vi "swingup_pendulum_energy.vi"(0 "alpha_full (rad)":dbl, 1 "alpha_dot (rad/s)":dbl, 2 "mp (kg)":dbl=0.027000000700354576 caption="Mp" min=0.0 step=0.0010000000474974513 format="%_3f", 3 "lp (m)":dbl=0.15299999713897705 caption="lp" min=0.0 max=1.0 step=0.0010000000474974513 format="%#_3f", 4 "Jp (kg.m^2)":dbl=0.00011999999696854502 caption="Jp" min=0.0 max=0.0010000000474974513 step=9.999999747378752e-06 format="%_3g") -> (5 "E (mJ)":dbl)   [LabVIEW 2021]
doc: "Calculates the total energy of a pendulum."
panel:
  # "Distance from pivot to CM"
  # "Moment of inertia about CM."
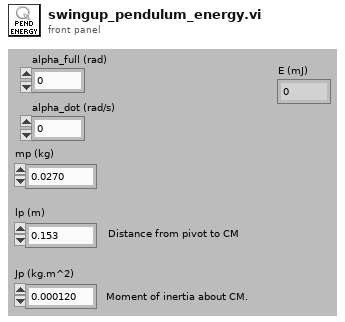
[diagram p1: front panel]
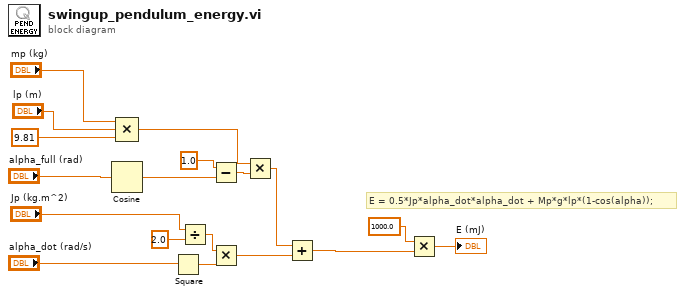
[diagram p0: block diagram]
diagram:
  # "E = 0.5*Jp*alpha_dot*alpha_dot + Mp*g*lp*(1-cos(alpha));"
  n1 = Cosine(x="alpha_full (rad)") -> (cos(x)=w11:dbl)
  n2 = Compound Arithmetic op=MULTIPLY("mp (kg)", "lp (m)", 9.81 ("value")) -> (w12:dbl)
  n3 = Square(x="alpha_dot (rad/s)") -> (x^2=w18:dbl)
  n4 = Divide(x="Jp (kg.m^2)", y=2.0) -> (x/y=w17:dbl)
  n5 = Subtract(x=1.0, y=w11) -> (x-y=w14:dbl)
  n6 = Multiply(x=w17, y=w18) -> (x*y=w16:dbl)
  n7 = Multiply(x=w12, y=w14) -> (x*y=w9:dbl)
  n8 = Add(x=w9, y=w16) -> (x+y=w1:dbl)
  n9 = Multiply(x=1000.0 ("y"), y=w1) -> (x*y=→"E (mJ)":dbl)
